vi "Laser Unit Test VI.vi"() -> ()   [LabVIEW 2018]
doc: "This example performs a serial port write and a serial port read. The parameters set for the serial port must match the parameters of the connected instrument or device. The VISA Configure Serial Port VI sets the configuration parameters. The front panel displays the controls used to configure the basic parameters, such as baud rate, data bits, and parity. The VI passes the VISA resource name to other VIs that perform operations on that VISA resource. The VISA Write function sends a command to the serial device and the VISA Read function returns data based on the command. The VISA Close function then closes the reference to the serial device. It is important to close the reference; otherwise, further communication through that port might not be possible."
uses:
  PPLs/Laser/Parent/Laser.lvlibp/Laser.lvclass
panel:
  out "Status":bool
  in  "Device":string="Laser"
  in  "PPLs Folder Path":path=path "C:/AME Test Engineering/LabVIEW/PPLs"
  in  "INI File Path":path=path "C:/Projects/Transceiver Boresight Station/Source/Station Configuration/config.ini"
  out "Error Out":errorcluster={"status"=TRUE, "code"=-43, "source"="File Path not found"}
  in  "Error In":errorcluster
  in  "stop":bool
  in  "Commands":string[](array[string])=["read-sn"]
  in  "Send Commands (non-enum)":bool
  out "Response":string="\r\n\r\n"
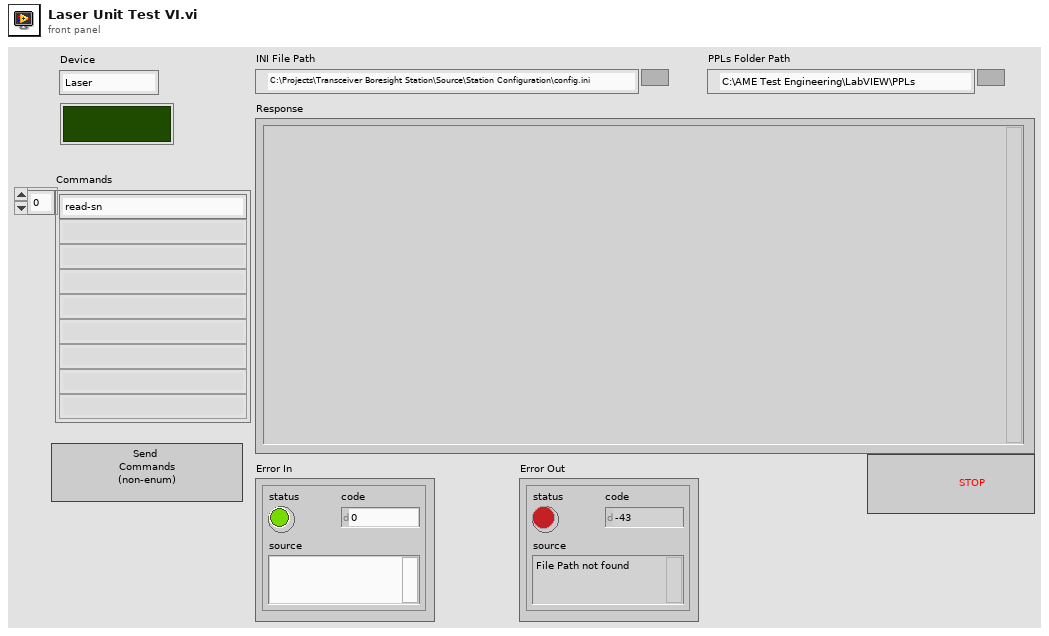
[diagram p1: front panel]
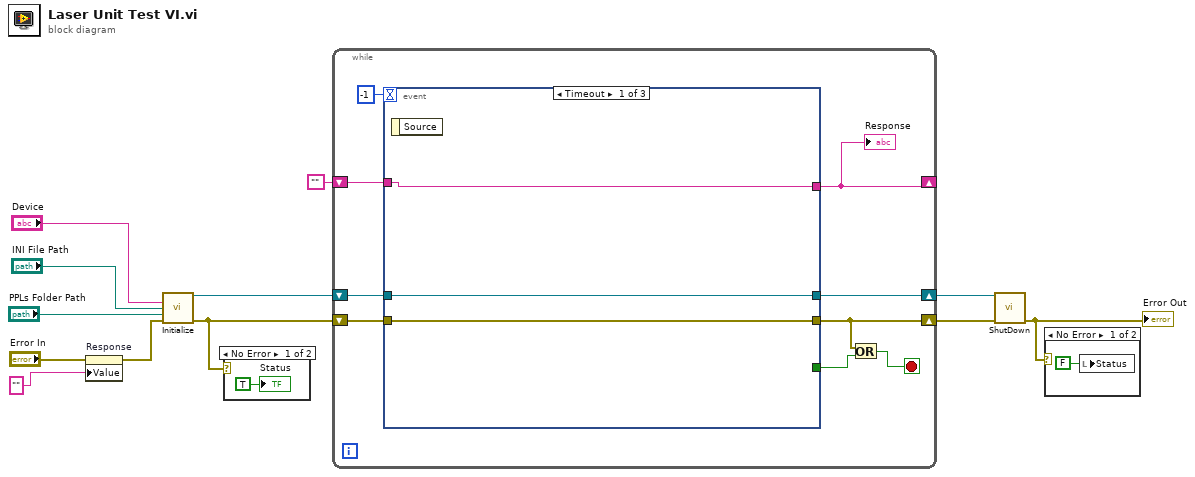
[diagram p0: block diagram]
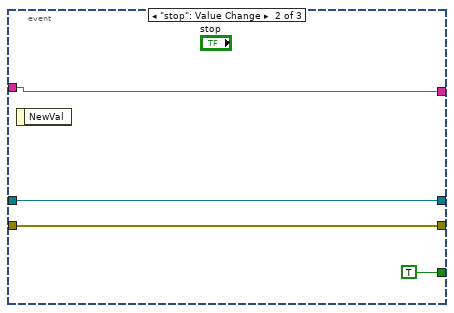
[diagram p4: hidden frame]
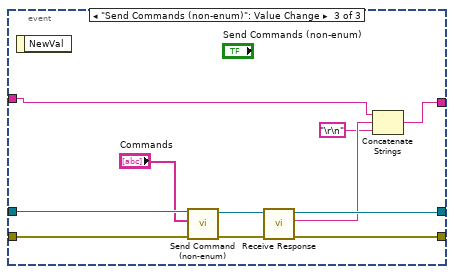
[diagram p5: hidden frame]
diagram:
  n1 = property on="Response" class="Str"(error in="Error In", "Value"="" ("Response")) -> (error out=w2:errorcluster)  [unwired: 1 in, 1 out]
  n2 = call "Initialize.vi"("Device"="Device", "INI File Path"="INI File Path", "PPLs Folder Path"="PPLs Folder Path", "error in"=w2) -> ("Laser out"=w9:refnum<class "Laser.lvclass">, "error out"=w5:errorcluster)  [unwired: 10 in]
  n3 = case shown="No Error" w5 {
    frame No Error {
      "Status" <- TRUE ("Status")
    }
    frame Error {
    }
  }
  n4 = while {
    shift-right: [w16] -> w7
    shift-left: w5 -> [w20]
    shift-right: [w19] -> w6
    shift-left: w9 -> [w21]
    shift-right: [w18] -> _
    shift-left: "" -> [w17]
    stop <- w14 stop-if-true
    n5 = event shown="[0] Timeout" {
      selector: _ -> [_ _ _]
      dyn-events: _ -> [_ _ _]
      timeout: -1 -> [_ _ _]
      tunnel: w21 -> [w25 w29 w40]
      tunnel: w20 -> [w24 w28 w38]
      tunnel: [w25 w29 w35] -> w19
      tunnel: [w24 w28 w34] -> w16
      tunnel: [w23 w26 w30] -> w18
      tunnel: w17 -> [w23 w26 w33]
      tunnel: [_ TRUE _] -> w15
      event Timeout {
        n6 = event-data() -> ()  [unwired: 1 in, 1 out]
      }
      event "stop": Value Change {
        n7 = event-data() -> ()  [unwired: 1 in, 1 out]
      }
      event "Send Commands (non-enum)": Value Change {
        n8 = event-data() -> ()  [unwired: 1 in, 1 out]
        n9 = call-dynamic "Send Command (non-enum).vi"("error in (no error)"=w38, "Commands"="Commands", "Laser in"=w40) -> ("error out"=w36:errorcluster, "Laser out"=w37:refnum<class "Laser.lvclass">)  [unwired: 7 in]
        n10 = call-dynamic "Receive Response.vi"("error in (no error)"=w36, "Laser in"=w37) -> ("error out"=w34:errorcluster, "Response"=w32:string, "Laser out"=w35:refnum<class "Laser.lvclass">)  [unwired: 7 in]
        n11 = Concatenate Strings(w33, w32, "\r\n") -> (w30:string)
      }
    }
    "Response" <- w18
    n12 = Or(x=w16, y=w15) -> (x .or. y?=w14:bool)
  }
  n13 = call "ShutDown.vi"("error in"=w7, "Laser in"=w6) -> ("error out"=w4:errorcluster)  [unwired: 8 in, 1 out]
  "Error Out" <- w4
  n14 = case shown="No Error" w4 {
    frame No Error {
      n15 = local write "Status"(FALSE ("Status")) -> ()
    }
    frame Error {
    }
  }
